vi "TestProgram1Keithley.vi"() -> ()   [LabVIEW 2014]
panel:
  out "Numeric":dbl
  in  "Configure":bool
  in  "Clear graph?":bool
  out "Resistance VS Temperature":cluster{dbl[], dbl[]}(graph)
  out "Byte Stream File Refnum":refnum<file>
  in  "file path (use dialog)":path
  out "Current Temperature":string
  out "Return":string
  in  "Set Temperature Command":string
  in  "Set Temperature":bool
  out "Return Value Temp":string
  in  "Command Temp":string
  in  "Temp":refnum<visa-resource-name>
  out "Return Value 1":string
  in  "Command  1":string
  in  "Multimeter 1":refnum<visa-resource-name>
  in  "Measure":bool
  in  "stop":bool
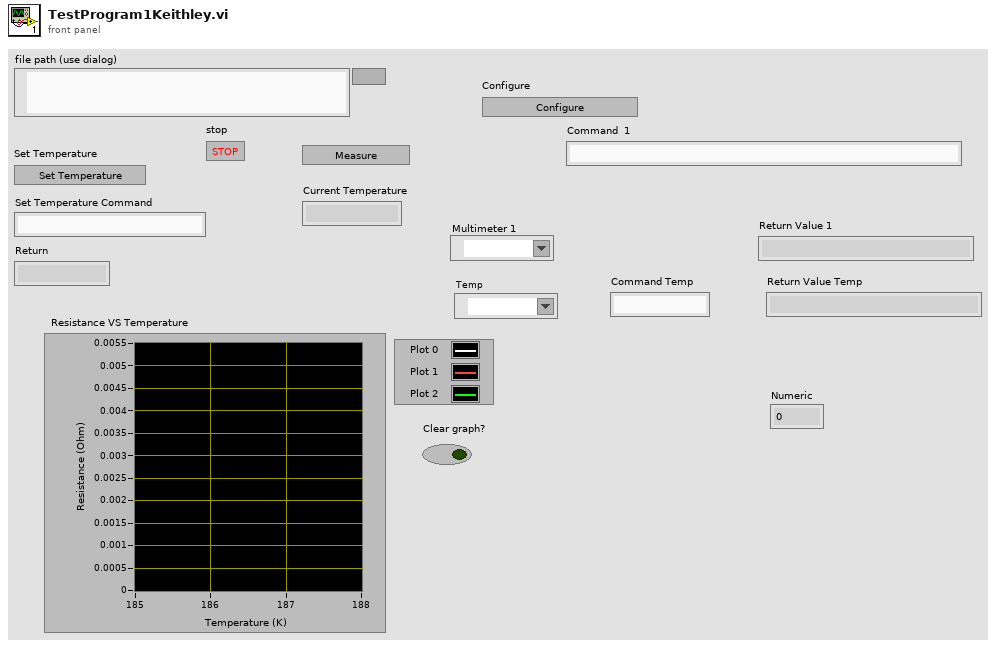
[diagram p1: front panel]
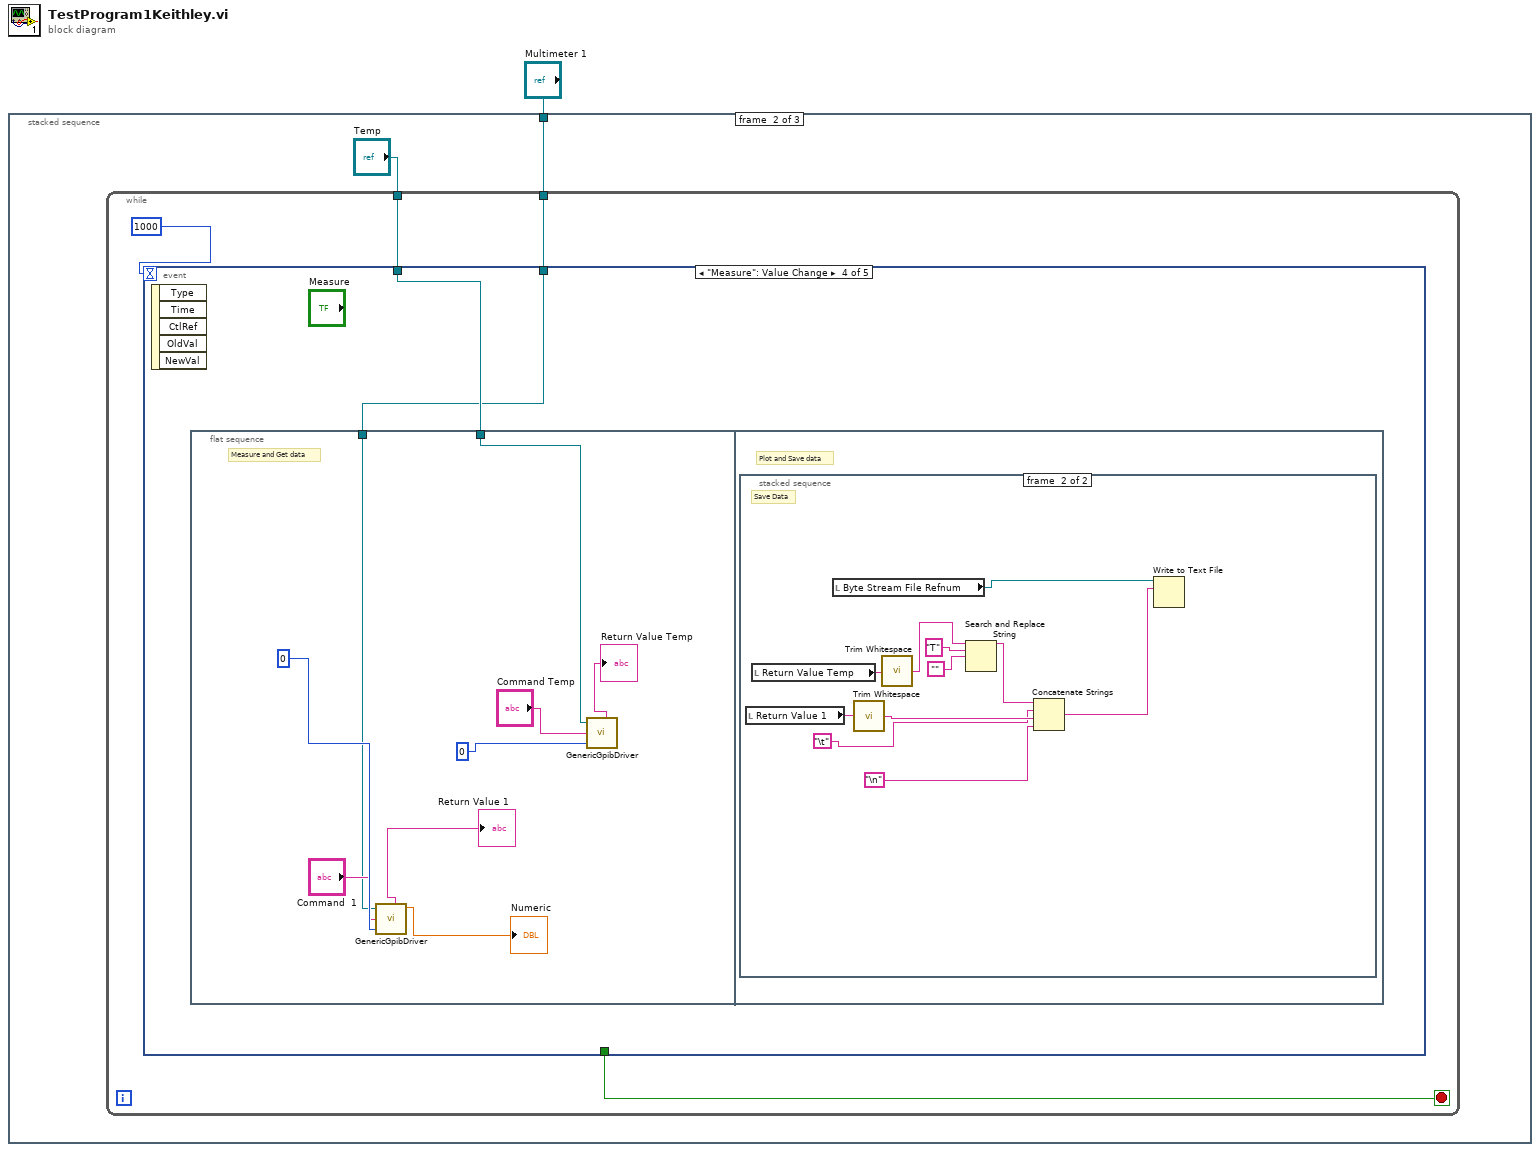
[diagram p0: block diagram]
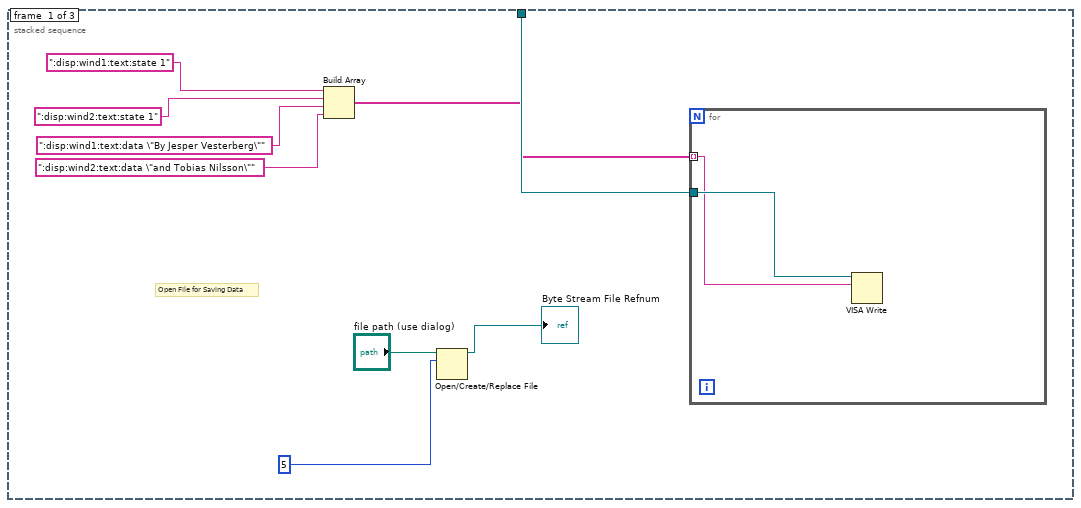
[diagram p2: hidden frame]
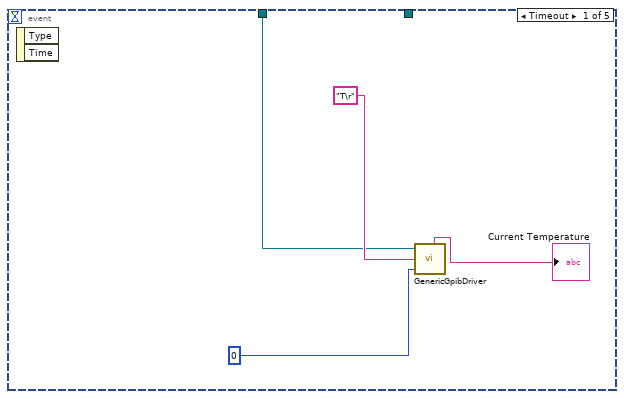
[diagram p3: hidden frame]
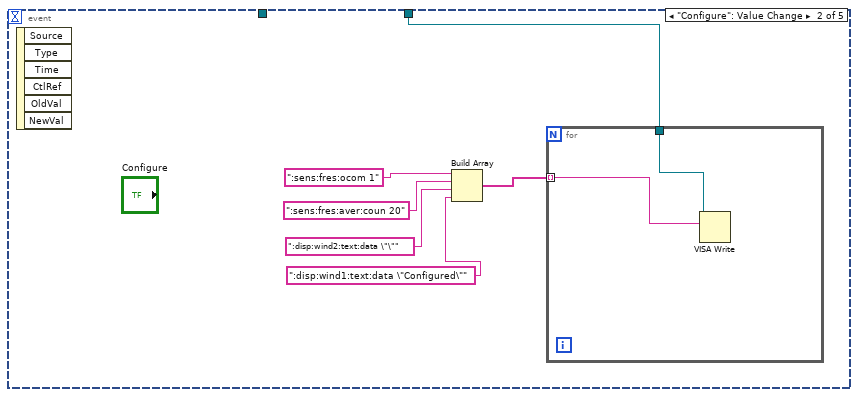
[diagram p4: hidden frame]
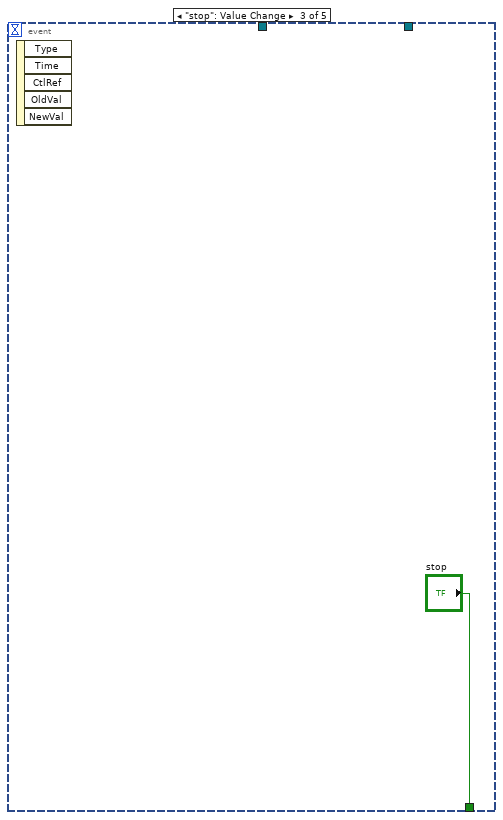
[diagram p5: hidden frame]
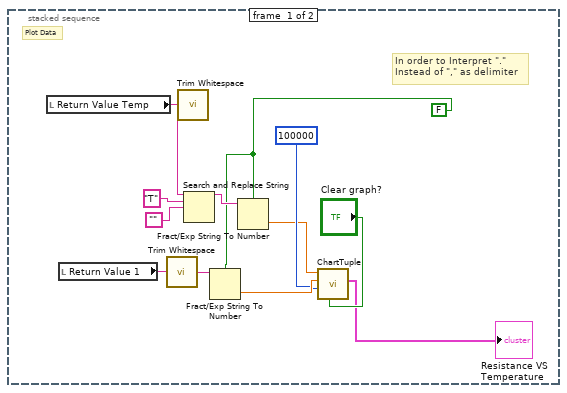
[diagram p6: hidden frame]
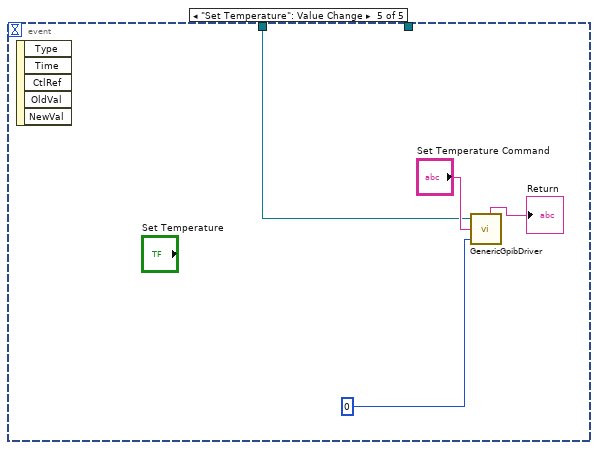
[diagram p7: hidden frame]
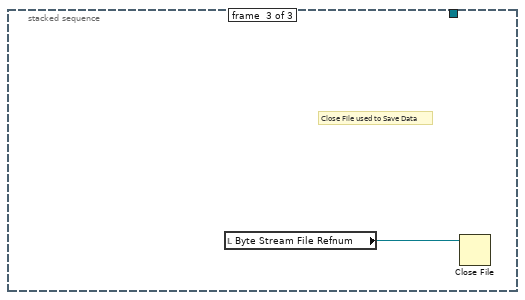
[diagram p8: hidden frame]
diagram:
  n1 = stacked-sequence {
    tunnel: "Multimeter 1" -> [w7 w13 _]
    frame #0 {
      # "Open File for Saving Data"
      n2 = Build Array(":disp:wind1:text:state 1", ":disp:wind2:text:state 1", ":disp:wind1:text:data \"By Jesper Vesterberg\"", ":disp:wind2:text:data \"and Tobias Nilsson\"") -> (w3:string[])
      n3 = Open/Create/Replace File(file path (use dialog)="file path (use dialog)", operation (0:open)=5) -> (refnum out=→"Byte Stream File Refnum":refnum<file>)  [unwired: 4 in, 2 out]
      n4 = for {
        tunnel: w7 -> [w12]
        tunnel: w3 -> [w11] mode=indexing
        n5 = VISA Write(VISA resource name=w12, write buffer=w11) -> ()  [unwired: 1 in, 3 out]
      }
    }
    frame #1 {
      n6 = while {
        tunnel: "Temp" -> [w17]
        tunnel: w13 -> [w15]
        stop <- w18 stop-if-true
        n7 = event shown="[3] \"Measure\": Value Change" {
          selector: _ -> [_ _ _ _ _]
          dyn-events: _ -> [_ _ _ _ _]
          timeout: 1000 -> [_ _ _ _ _]
          tunnel: [_ _ "stop" _ _] -> w18
          tunnel: w17 -> [w21 _ _ w33 w68]
          tunnel: w15 -> [_ w25 _ w32 _]
          event Timeout {
            n8 = event-data() -> ()  [unwired: 1 in, 2 out]
            n9 = call "GenericGpibDriver.vi"("Wait (ms)"=0, "Command"="T\r", "VISA resource name"=w21) -> ("Return Value"=→"Current Temperature":string)  [unwired: 1 in, 4 out]
          }
          event "Configure": Value Change {
            n10 = event-data() -> ()  [unwired: 1 in, 6 out]
            n11 = Build Array(":sens:fres:ocom 1", ":sens:fres:aver:coun 20", ":disp:wind2:text:data \"\"", ":disp:wind1:text:data \"Configured\"") -> (w26:string[])
            n12 = for {
              tunnel: w26 -> [w30] mode=indexing
              tunnel: w25 -> [w29]
              n13 = VISA Write(VISA resource name=w29, write buffer=w30) -> ()  [unwired: 1 in, 3 out]
            }
          }
          event "stop": Value Change {
            n14 = event-data() -> ()  [unwired: 1 in, 5 out]
          }
          event "Measure": Value Change {
            n15 = event-data() -> ()  [unwired: 1 in, 5 out]
            n16 = flat-sequence {
              tunnel: w33 -> [w36]
              tunnel: w32 -> [w37]
              frame #0 {
                # "Measure and Get data"
                n17 = call "GenericGpibDriver.vi"("Wait (ms)"=0, "Command"="Command  1", "VISA resource name"=w37) -> ("Return Value"=→"Return Value 1":string, "Bytes Read"=→"Numeric":dbl)  [unwired: 1 in, 3 out]
                n18 = call "GenericGpibDriver.vi"("Wait (ms)"=0, "Command"="Command Temp", "VISA resource name"=w36) -> ("Return Value"=→"Return Value Temp":string)  [unwired: 1 in, 4 out]
              }
              frame #1 {
                # "Plot and Save data"
                n19 = stacked-sequence {
                  frame #0 {
                    w45 = FALSE
                    # "In order to Interpret \".\" \nInstead of \",\" as delimiter"
                    # "Plot Data"
                    n20 = local read "Return Value Temp"() -> (w52:string)
                    n21 = local read "Return Value 1"() -> (w51:string)
                    n22 = call <vilib>:"Trim Whitespace.vi"("string"=w51) -> ("trimmed string"=w49:string)  [unwired: 1 in]
                    n23 = call <vilib>:"Trim Whitespace.vi"("string"=w52) -> ("trimmed string"=w50:string)  [unwired: 1 in]
                    n24 = Search and Replace String(input string=w50, search string="T", replace string="") -> (result string=w53:string)  [unwired: 5 in, 3 out]
                    n25 = Fract/Exp String To Number(use system decimal point (T)=w45, string=w49) -> (number=w48:dbl)  [unwired: 2 in, 1 out]
                    n26 = Fract/Exp String To Number(use system decimal point (T)=w45, string=w53) -> (number=w46:dbl)  [unwired: 2 in, 1 out]
                    n27 = call "ChartTuple.vi"("Clear Graph?"="Clear graph?", "Chart History (10,000)"=100000, "Y Value"=w48, "X Value"=w46) -> ("XY Graph"=→"Resistance VS Temperature":cluster{dbl[], dbl[]})  [unwired: 7 in]
                  }
                  frame #1 {
                    # "Save Data"
                    n28 = local read "Return Value 1"() -> (w63:string)
                    n29 = local read "Return Value Temp"() -> (w64:string)
                    n30 = local read "Byte Stream File Refnum"() -> (w65:refnum<file>)
                    n31 = call <vilib>:"Trim Whitespace.vi"("string"=w63) -> ("trimmed string"=w62:string)  [unwired: 1 in]
                    n32 = call <vilib>:"Trim Whitespace.vi"("string"=w64) -> ("trimmed string"=w59:string)  [unwired: 1 in]
                    n33 = Search and Replace String(input string=w59, search string="T", replace string="") -> (result string=w58:string)  [unwired: 5 in, 3 out]
                    n34 = Concatenate Strings(w58, "\t", w62, "\n") -> (w66:string)
                    n35 = Write to Text File(file (use dialog)=w65, text=w66) -> ()  [unwired: 2 in, 3 out]
                  }
                }
              }
            }
          }
          event "Set Temperature": Value Change {
            n36 = event-data() -> ()  [unwired: 1 in, 5 out]
            n37 = call "GenericGpibDriver.vi"("Wait (ms)"=0, "Command"="Set Temperature Command", "VISA resource name"=w68) -> ("Return Value"=→"Return":string)  [unwired: 1 in, 4 out]
          }
        }
      }
    }
    frame #2 {
      # "Close File used to Save Data"
      n38 = local read "Byte Stream File Refnum"() -> (w71:refnum<file>)
      n39 = Close File(refnum=w71) -> ()  [unwired: 1 in, 2 out]
    }
  }
